vi "GDSFile_FindPrefix.vi"(1 "Filenames as references":string[](array[string]), 3 "Filenames to search":string[](array[string]), 5 "error in (no error)":errorcluster) -> (15 "Prefix":string, 17 "Separator":string, 19 "error out":errorcluster)   [LabVIEW 2020]
doc: "Finds the common prefix in a list of file names. Empty string elements are ignored."
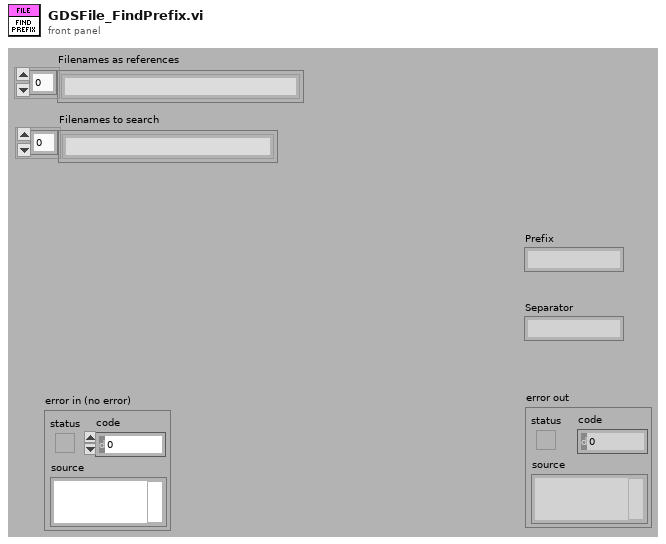
[diagram p1: front panel]
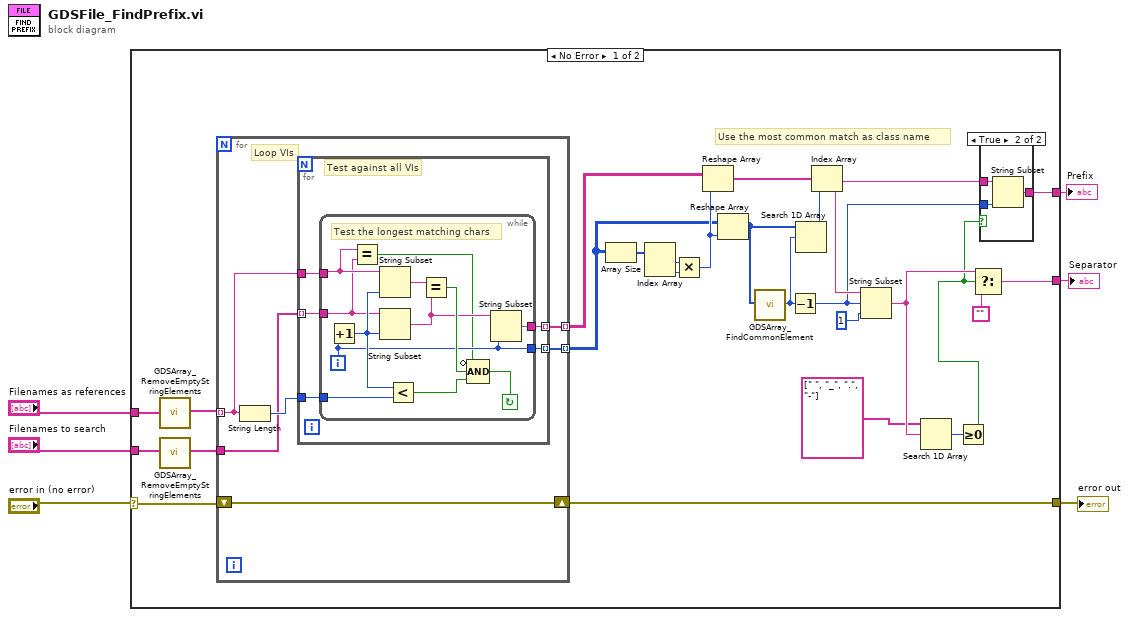
[diagram p0: block diagram]
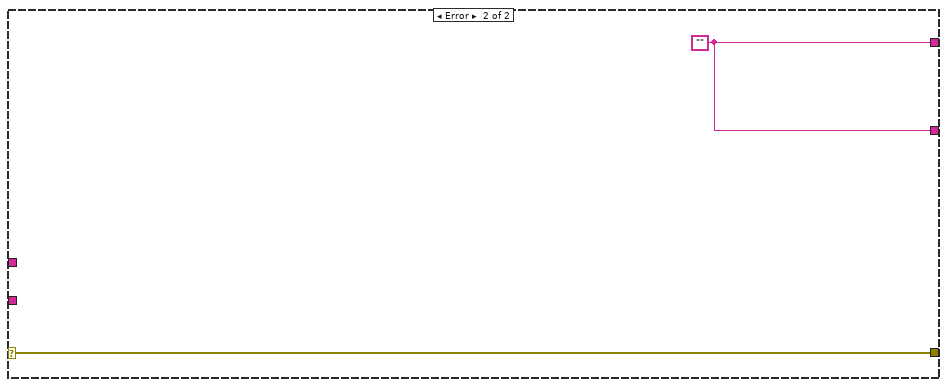
[diagram p3: hidden frame]
diagram:
  n1 = case shown="No Error" "error in (no error)" {
    selector: "error in (no error)" -> [w15 w61]
    tunnel: [w18 w60] -> w6
    tunnel: [w17 w60] -> w5
    tunnel: "Filenames as references" -> [w14 _]
    tunnel: "Filenames to search" -> [w12 _]
    tunnel: [w16 w61] -> w4
    frame No Error {
      # "Use the most common match as class name"
      n2 = call <resource>:"GDSArray_RemoveEmptyStringElements.vi"("String array"=w14) -> ("String array out"=w13:string[])  [unwired: 18 in]
      n3 = call <resource>:"GDSArray_RemoveEmptyStringElements.vi"("String array"=w12) -> ("String array out"=w11:string[])  [unwired: 18 in]
      n4 = for {
        shift-right: [w38] -> w16
        shift-left: w15 -> [w38]
        tunnel: w13 -> [w41] mode=indexing
        tunnel: [w39] -> w19 mode=indexing
        tunnel: [w40] -> w20 mode=indexing
        tunnel: w11 -> [w37]
        # "Loop VIs"
        n5 = String Length(string=w41) -> (length=w42:i32)
        n6 = for {
          tunnel: w37 -> [w47] mode=indexing
          tunnel: w42 -> [w46]
          tunnel: w41 -> [w45]
          tunnel: [w44] -> w40 mode=indexing
          tunnel: [w43] -> w39 mode=indexing
          # "Test against all VIs"
          n7 = while {
            tunnel: [w51] -> w44
            tunnel: [w53] -> w43
            tunnel: w45 -> [w50]
            tunnel: w46 -> [w57]
            tunnel: w47 -> [w49]
            i -> [w53]
            stop <- w58 continue-if-true
            # "Test the longest matching chars"
            n8 = Increment(x=w53) -> (x+1=w56:i32)
            n9 = Equal?(x=w50, y=w49) -> (x = y?=w48:bool)
            n10 = String Subset(string=w50, length (rest)=w56) -> (substring=w55:string)  [unwired: 1 in]
            n11 = String Subset(string=w49, length (rest)=w56) -> (substring=w52:string)  [unwired: 1 in]
            n12 = Less?(x=w56, y=w57) -> (x < y?=w59:bool)
            n13 = Equal?(x=w55, y=w52) -> (x = y?=w54:bool)
            n14 = Compound Arithmetic op=AND(invert w48, w54, w59) -> (w58:bool)
            n15 = String Subset(string=w52, length (rest)=w53) -> (substring=w51:string)  [unwired: 1 in]
          }
        }
      }
      n16 = Array Size(array=w19) -> (size(s)=w32:i32[])
      n17 = Index Array(array=w32) -> (element #1=w30:i32, element #2=w31:i32)  [unwired: 2 in]
      n18 = Multiply(x=w30, y=w31) -> (x*y=w28:i32)
      n19 = Reshape Array(w20, w28) -> (w25:string[])
      n20 = Reshape Array(w19, w28) -> (w26:i32[])
      n21 = call <resource>:"GDSArray_FindCommonElement.vi"("I32Array"=w26) -> ("MostCommonElement"=w27:i32)  [unwired: 17 in, 1 out]
      n22 = Decrement(x=w27) -> (x-1=w21:i32)
      n23 = Search 1D Array(1D array=w26, element=w27) -> (index of element=w24:i32)  [unwired: 1 in]
      n24 = Index Array(array=w25, index=w24) -> (element=w22:string)
      n25 = String Subset(string=w22, offset (0)=w21, length (rest)=1 ("length (rest)")) -> (substring=w10:string)
      n26 = Search 1D Array(1D array=string[] [" ", "_", ".", "-"], element=w10) -> (index of element=w8:i32)  [unwired: 1 in]
      n27 = Greater Or Equal To 0?(x=w8) -> (x >= 0?=w7:bool)
      n28 = Select(t=w10, s=w7, f="") -> (s? t:f=w17:string)
      n29 = case shown="True" w7 {
        tunnel: w22 -> [w33 w36]
        tunnel: w21 -> [_ w35]
        tunnel: [w33 w34] -> w18
        frame False {
        }
        frame True {
          n30 = String Subset(string=w36, length (rest)=w35) -> (substring=w34:string)  [unwired: 1 in]
        }
      }
    }
    frame Error {
      w60 = ""
    }
  }
  "Prefix" <- w6
  "Separator" <- w5
  "error out" <- w4
